vi "Send To Created.vi"(4 "Is Priority":bool, 6 "Alias":string, 10 "Msg":refnum<class "Msg.lvclass">, 11 "Base Actor in":refnum<class "Base Actor.lvclass">) -> (0 "Error out":errorcluster)   [LabVIEW 2025, in "jettl.lvlib" / "Actor.lvlib" / "Base Actor.lvclass"]
uses:
  Base Actor.lvclass
  Msg/Msg.lvclass
  Relation.ctl
  Attributes/Attributes/Attributes.lvclass
  Base Actor.lvclass/Base Actor.ctl
  Actor.lvlib
  Error/Error.lvlib
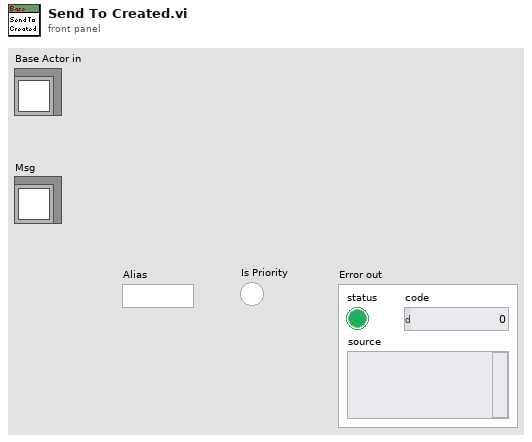
[diagram p1: front panel]
types:
  T1 = typedef "jettl.lvlib/Actor.lvlib/Relation.ctl" = enum16{"Self", "Creator", "Created"}
  T2 = typedef "jettl.lvlib/Actor.lvlib/Msg Set.ctl" = set{refnum<class "Msg.lvclass">}
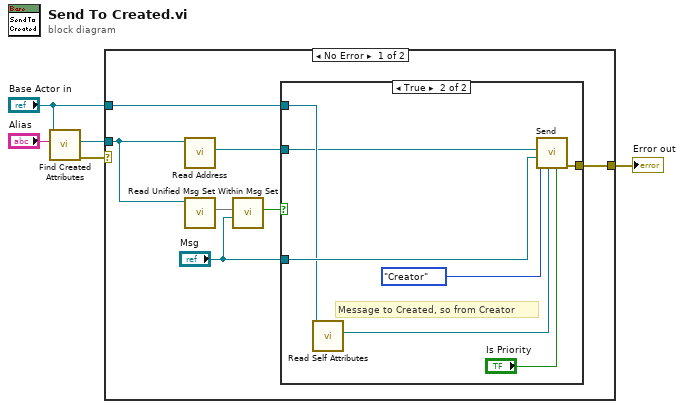
[diagram p0: block diagram]
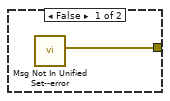
[diagram p2: hidden frame]
diagram:
  n1 = call-dynamic "Find Created Attributes.vi"("Alias"="Alias", "Base Actor in"="Base Actor in") -> ("Error out"=w2:errorcluster, "Created Attributes"=w1:refnum<class "Attributes.lvclass">)  [unwired: 8 in]
  n2 = case shown="No Error" w2 {
    selector: w2 -> [_ w21]
    tunnel: "Base Actor in" -> [w7 _]
    tunnel: [w12 w21] -> w5
    tunnel: w1 -> [w6 _]
    frame No Error {
      n3 = call-dynamic "Read Address.vi"("Attributes in"=w6) -> ("Address"=w9:refnum<user-event>)  [unwired: 10 in]
      n4 = call-dynamic "Read Unified Msg Set.vi"("Attributes in"=w6) -> ("Unified Msg Set"=w11:T2)  [unwired: 10 in]
      n5 = call "Within Msg Set.vi"("Msg"="Msg", "Msg Set"=w11) -> ("Within Msg Set"=w10:bool)  [unwired: 9 in]
      n6 = case shown="True" w10 {
        tunnel: w7 -> [_ w16]
        tunnel: "Msg" -> [_ w20]
        tunnel: [w13 w15] -> w12
        tunnel: w9 -> [_ w14]
        frame False {
          n7 = call "Msg Not In Unified Set--error.vi"() -> ("Error"=w13:errorcluster)  [unwired: 11 in]
        }
        frame True {
          # "Message to Created, so from Creator"
          n8 = call-dynamic "Read Self Attributes.vi"("Base Actor in"=w16) -> ("Self Attributes"=w18:refnum<class "Attributes.lvclass">)  [unwired: 10 in]
          n9 = call "Send.vi"("Is Priority"="Is Priority", "Self Attributes"=w18, "Relation"=Relation."Creator", "Msg"=w20, "Address"=w14) -> ("Error out"=w15:errorcluster)  [unwired: 6 in]
        }
      }
    }
    frame Error {
    }
  }
  "Error out" <- w5
